vi "Create ByteArray Content.vi"(5 "HttpContent_String in":refnum<class "HttpContent_ByteArray.lvclass">, 8 "error in (no error)":errorcluster, 11 "content":u8[](array[numeric])) -> (0 "error out":errorcluster, 3 "HttpContent_String out":refnum<class "HttpContent_ByteArray.lvclass">)   [LabVIEW 2018, in "HttpClient_NET.lvlib" / "HttpContent_ByteArray.lvclass"]
doc: "<b> </b> <b> </b>\nHttpClient_NET\nJustin Young - Viviota\nCopyright (c) 2021\nLicense: BSD"
uses:
  HttpContent_ByteArray.lvclass
  C:/Viviota/Projects/R&D/LabVIEW_HTTP_REST_NET/HttpContent/HttpContent.lvclass
  System.Net.Http
  HttpContent/HttpContent.lvclass
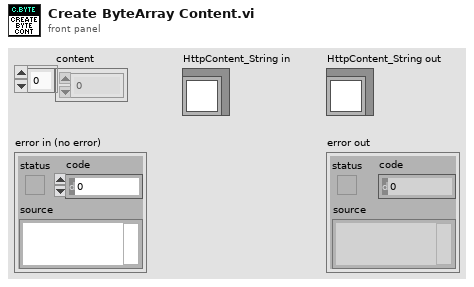
[diagram p1: front panel]
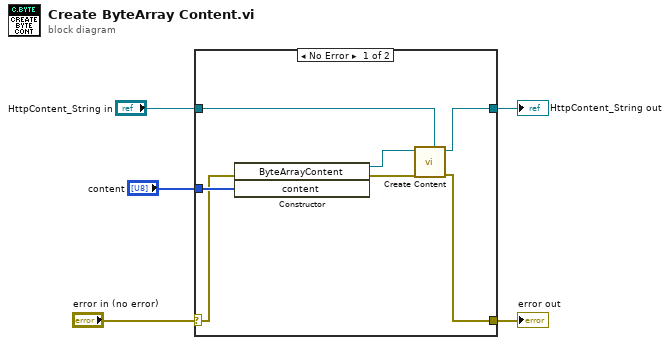
[diagram p0: block diagram]
diagram:
  n1 = case shown="No Error" "error in (no error)" {
    selector: "error in (no error)" -> [w7 w14]
    tunnel: [w6 w14] -> w4
    tunnel: [w11 w13] -> w2
    tunnel: "HttpContent_String in" -> [w12 w13]
    tunnel: "content" -> [w8 _]
    frame No Error {
      n2 = constructor class="ByteArrayContent"(error in=w7, "content"=w8) -> (reference out=w9:refnum<k24>, error out=w10:errorcluster)  [unwired: 2 in, 2 out]
      n3 = call "Create Content.vi"("HttpContent in"=w12, "error in (no error)"=w10, "NET_HttpContent"=w9) -> ("error out"=w6:errorcluster, "HttpContent out"=w11:refnum<class "HttpContent_ByteArray.lvclass">)  [unwired: 7 in]
    }
    frame Error {
    }
  }
  "error out" <- w4
  "HttpContent_String out" <- w2
